vi "Excercise 3-8.vi"() -> ()   [LabVIEW 2014]
panel:
  out "Warning?":bool
  out "Warning Text":string
  in  "Min Temp":dbl
  in  "Max Temp":dbl
  in  "Current Temp":dbl
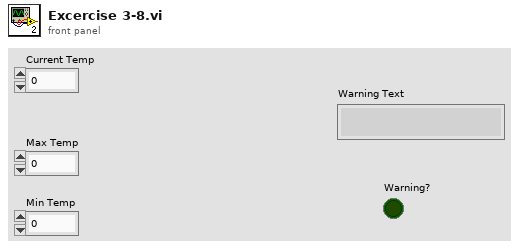
[diagram p1: front panel]
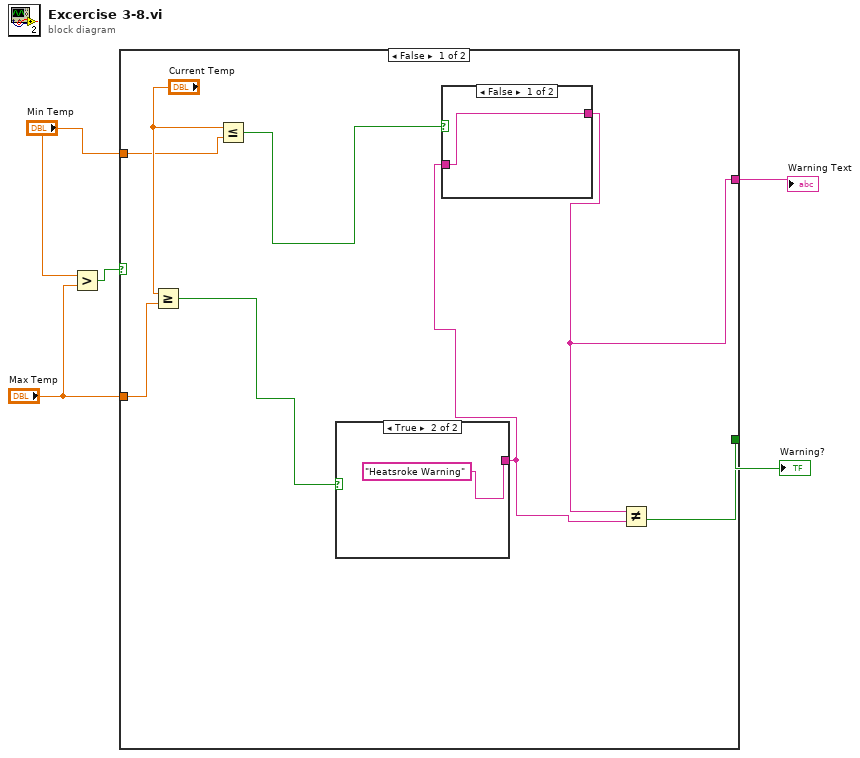
[diagram p0: block diagram]
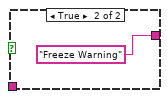
[diagram p2: hidden frame]
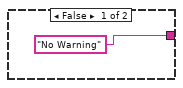
[diagram p3: hidden frame]
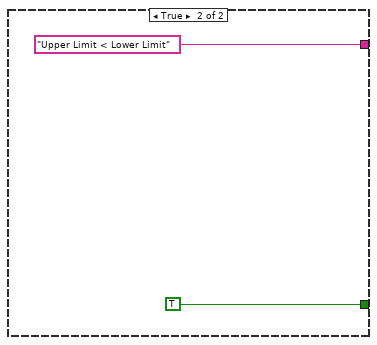
[diagram p4: hidden frame]
diagram:
  n1 = Greater?(x="Min Temp", y="Max Temp") -> (0:w1:bool)
  n2 = case shown="False" w1 {
    tunnel: [w12 TRUE] -> w5
    tunnel: [w6 "Upper Limit < Lower Limit"] -> w4
    tunnel: "Min Temp" -> [w11 _]
    tunnel: "Max Temp" -> [w10 _]
    frame False {
      n3 = Greater Or Equal?(x="Current Temp", y=w10) -> (x >= y?=w9:bool)
      n4 = Less Or Equal?(x="Current Temp", y=w11) -> (x <= y?=w8:bool)
      n5 = case shown="True" w9 {
        tunnel: ["No Warning" "Heatsroke Warning"] -> w7
        frame False {
        }
        frame True {
        }
      }
      n6 = case shown="False" w8 {
        tunnel: [w14 "Freeze Warning"] -> w6
        tunnel: w7 -> [w14 _]
        frame False {
        }
        frame True {
        }
      }
      n7 = Not Equal?(x=w6, y=w7) -> (x != y?=w12:bool)
    }
    frame True {
    }
  }
  "Warning Text" <- w4
  "Warning?" <- w5
